vi "Destroy.vi"(8 "error in (no error)":errorcluster, 11 "CIFFIFO in":refnum<class "CIF_NIChn_Fifo_U8.lvclass">) -> (0 "error out":errorcluster, 3 "CIFFIFO out":refnum<class "CIF_NIChn_Fifo_U8.lvclass">)   [LabVIEW 2021, in "CIF_NIChn_Fifo_U8.lvclass"]
uses:
  CIF_NIChn_Fifo_U8.lvclass
  CIF_NIChn_Fifo_U8.lvclass/CIF_NIChn_Fifo_U8.ctl
  <vilib>/CIF Foundation/NI Channels/NIChannels.lvlib
  NIChn/CIF_NIChn.lvclass
  D:/dev/Packages/Channel_Manager/src/CIF_NIChn/NIChn/CIF_NIChn.lvclass
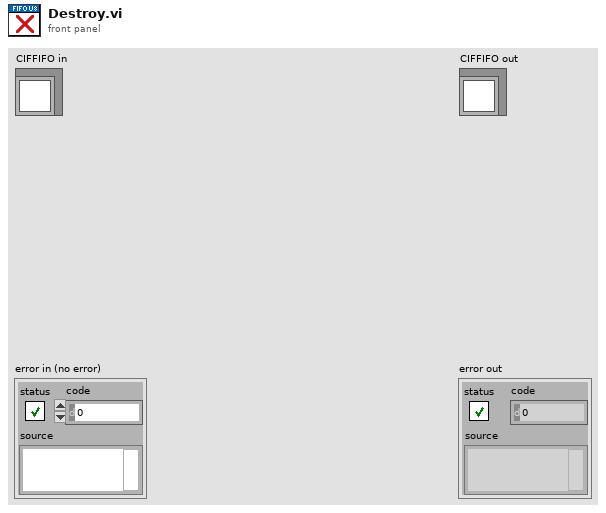
[diagram p1: front panel]
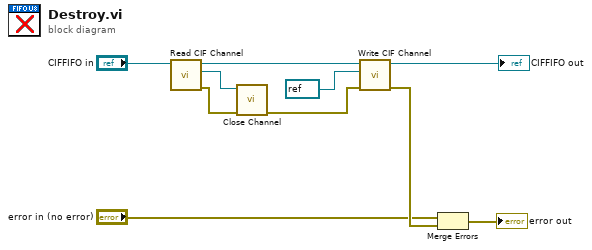
[diagram p0: block diagram]
diagram:
  n1 = call "Read CIF Channel.vi"("CIFTag in"="CIFFIFO in") -> ("error out"=w5:errorcluster, "CIF Channel"=w9:refnum<k21>, "CIFTag out"=w7:refnum<class "CIF_NIChn_Fifo_U8.lvclass">)  [unwired: 8 in]
  n2 = call <vilib>:"Close Channel.vi"("error in"=w5, "CIF Channel"=w9) -> ("error out"=w6:errorcluster)  [unwired: 9 in]
  n3 = call "Write CIF Channel.vi"("error in (no error)"=w6, "CIF Channel"=refnum<k21> refnum, "CIFTag in"=w7) -> ("error out"=w4:errorcluster, "CIFTag out"=→"CIFFIFO out":refnum<class "CIF_NIChn_Fifo_U8.lvclass">)  [unwired: 7 in]
  n4 = Merge Errors("error in (no error)", w4) -> (→"error out":errorcluster)
